vi "test pump.vi"() -> ()   [LabVIEW 2019]
panel:
  in  "Boolean":bool
  out "output value 2":dbl
  in  "Set Points 2":dbl[](array[numeric])=[23.0, 1.0, 167.0, 1.0, 2.0]
  in  "State":i16
  out "output value":dbl
  out "x/y":dbl
  out "Numeric":i32
  in  "stop":bool
  in  "Set Points":dbl[](array[numeric])=[23.0, 1.0, 167.0, 1.0, 2.0]
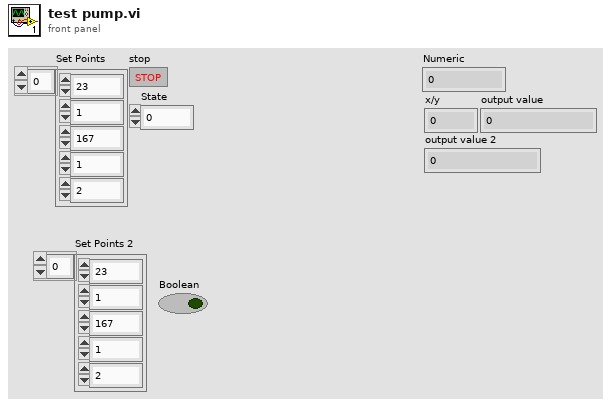
[diagram p1: front panel]
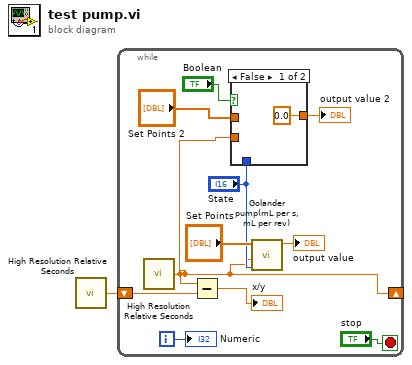
[diagram p0: block diagram]
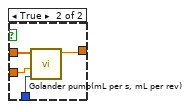
[diagram p2: hidden frame]
diagram:
  n1 = call <vilib>:"High Resolution Relative Seconds.vi"() -> ("relative seconds"=w1:dbl)
  n2 = while {
    shift-right: [w3] -> _
    shift-left: w1 -> [w10]
    i -> [w9]
    stop <- "stop" stop-if-true
    n3 = call <vilib>:"High Resolution Relative Seconds.vi"() -> ("relative seconds"=w3:dbl)
    n4 = Subtract(x=w3, y=w10) -> (x-y=→"x/y":dbl)
    n5 = case shown="False" "Boolean" {
      tunnel: "State" -> [_ w17]
      tunnel: [0.0 ("output value") w16] -> w5
      tunnel: "Set Points 2" -> [_ w15]
      tunnel: w3 -> [_ w14]
      frame False {
      }
      frame True {
        n6 = call "Golander pump(mL per s, mL per rev).vi"("State"=w17, "Time"=w14, "Set Points"=w15) -> ("output value"=w16:dbl)  [unwired: 3 in, 1 out]
      }
    }
    "output value 2" <- w5
    n7 = call "Golander pump(mL per s, mL per rev).vi"("State"="State", "Time"=w3, "Set Points"="Set Points") -> ("output value"=→"output value":dbl)  [unwired: 3 in, 1 out]
    "Numeric" <- w9
  }
